vi "ao_waveform_pc_infinite.vi"() -> ()   [LabVIEW 2020]
uses:
  <vilib>/measure/NI_MABase.lvlib
panel:
  out "x-y":u32
  out "Rounds":i32
  out "error out":errorcluster caption="错误输出"
  in  "停止":bool
  out "波形图":waveform(dbl)(graph)
  in  "SamplePeriod (ns)":u32=10000
  in  "Chan":u8
  in  "DevIndex":i32
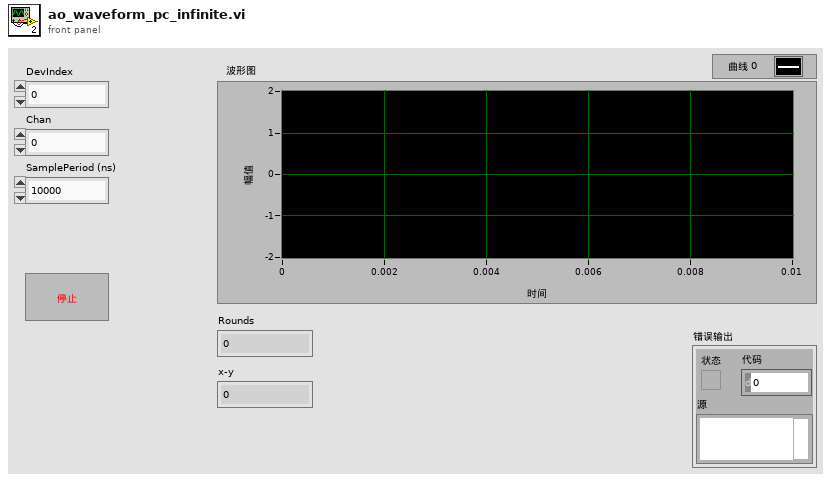
[diagram p1: front panel]
types:
  T1 = enum16{"Sine Wave", "Triangle Wave", "Square Wave", "Sawtooth Wave"}
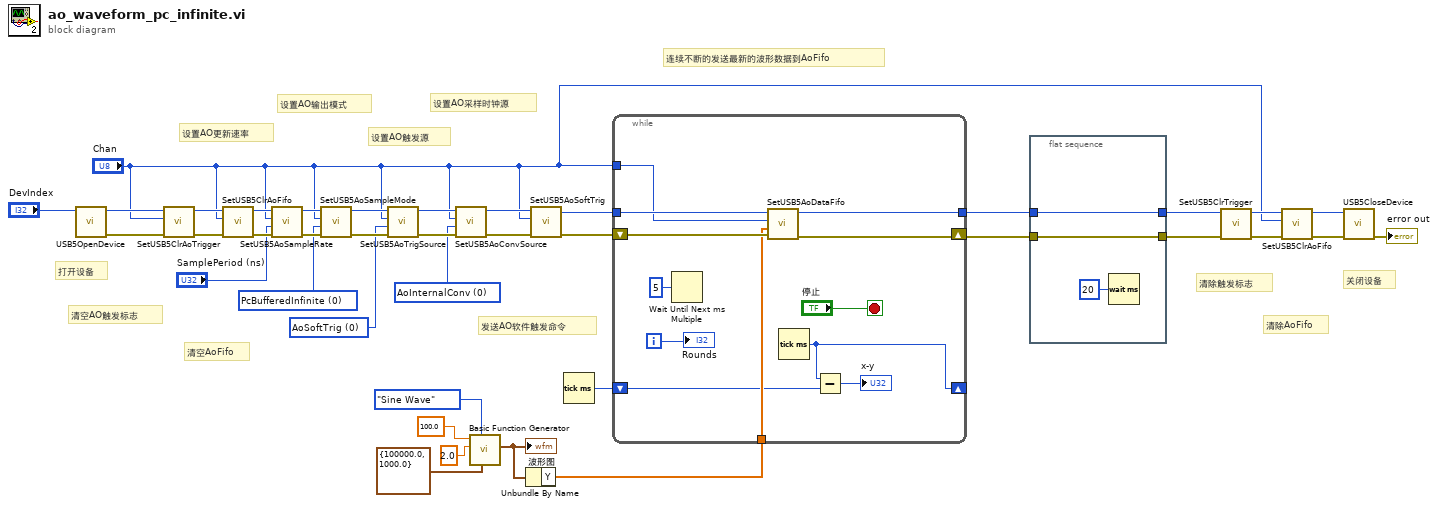
[diagram p0: block diagram]
diagram:
  w1 = u8 0 items=["AoInternalConv", "ConvIn", "AiConv", "DiConv", "DoConv", "Ao0Conv", "Ao1Conv", "Ao2Conv", "Ao3Conv"] ("AoConvSource")
  w2 = u8 0 items=["AoSoftTrig"=0, "ExtTrigIn"=1, "Din0RisingEdge"=2, "Din1RisingEdge"=3, "Din2RisingEdge"=4, "Din3RisingEdge"=5, "WithAiTrig"=6, "WithDiTrig"=7, "WithDoTrig"=8, "WithAo0Trig"=9, "WithAo1Trig"=10, "WithAo2Trig"=11, "WithAo3Trig"=12, "GlobalSoftTrig"=255] ("AoTrigSource")
  w3 = u8 0 items=["PcBufferedInfinite", "NCycle"] ("SampleMode")
  # "关闭设备"
  # "清除AoFifo"
  # "清除触发标志"
  # "连续不断的发送最新的波形数据到AoFifo"
  # "发送AO软件触发命令"
  # "设置AO采样时钟源"
  # "设置AO触发源"
  # "设置AO输出模式"
  # "设置AO更新速率"
  # "清空AoFifo"
  # "清空AO触发标志"
  # "打开设备"
  n1 = call "USB5OpenDevice.vi"("DevIndex"="DevIndex") -> ("error out"=w14:errorcluster, "DevIndex Out"=w15:i32)  [unwired: 9 in]
  n2 = call "SetUSB5ClrAoTrigger.vi"("错误输入（无错误）"=w14, "Chan"="Chan", "DevIndex"=w15) -> ("错误输出"=w12:errorcluster, "DevIndex Out"=w13:i32)  [unwired: 7 in]
  n3 = call "SetUSB5ClrAoFifo.vi"("错误输入（无错误）"=w12, "Chan"="Chan", "DevIndex"=w13) -> ("错误输出"=w32:errorcluster, "DevIndex Out"=w31:i32)  [unwired: 7 in]
  n4 = call "SetUSB5AoSampleRate.vi"("错误输入（无错误）"=w32, "SamplePeriod(ns)"="SamplePeriod (ns)", "Chan"="Chan", "DevIndex"=w31) -> ("错误输出"=w27:errorcluster, "DevIndex Out"=w28:i32)  [unwired: 6 in]
  n5 = call "SetUSB5AoSampleMode.vi"("错误输入（无错误）"=w27, "SampleMode"=w3, "Chan"="Chan", "DevIndex"=w28) -> ("错误输出"=w10:errorcluster, "DevIndex Out"=w11:i32)  [unwired: 6 in]
  n6 = call "SetUSB5AoTrigSource.vi"("错误输入（无错误）"=w10, "AoTrigSource"=w2, "Chan"="Chan", "DevIndex"=w11) -> ("错误输出"=w8:errorcluster, "DevIndex Out"=w9:i32)  [unwired: 6 in]
  n7 = call "SetUSB5AoConvSource.vi"("错误输入（无错误）"=w8, "AoConvSource"=w1, "Chan"="Chan", "DevIndex"=w9) -> ("错误输出"=w6:errorcluster, "DevIndex Out"=w7:i32)  [unwired: 6 in]
  n8 = call <vilib>:"Basic Function Generator.vi"("sampling info"=cluster{"Fs":dbl, "#s":dbl} {"Fs"=100000.0, "#s"=1000.0}, "signal type"=T1."Sine Wave", "amplitude"=2.0, "frequency"=100.0) -> ("signal out"=w34:waveform(dbl))  [unwired: 5 in, 2 out]
  "波形图" <- w34
  n9 = Unbundle By Name(w34) -> ("Y"=w33:dbl[])
  n10 = call "SetUSB5AoSoftTrig.vi"("错误输入（无错误）"=w6, "Chan"="Chan", "DevIndex"=w7) -> ("错误输出"=w25:errorcluster, "DevIndex Out"=w26:i32)  [unwired: 7 in]
  n11 = Tick Count (ms)() -> (millisecond timer value=w4:u32)
  n12 = while {
    tunnel: w26 -> [w50]
    tunnel: "Chan" -> [w48]
    tunnel: w33 -> [w46]
    tunnel: [w44] -> w18
    shift-right: [w43] -> w16
    shift-left: w25 -> [w49]
    shift-right: [w39] -> _
    shift-left: w4 -> [w41]
    i -> [w42]
    stop <- "停止" stop-if-true
    n13 = Wait Until Next ms Multiple(millisecond multiple=u32 5 ("毫秒倍数")) -> ()  [unwired: 1 out]
    n14 = call "SetUSB5AoDataFifo.vi"("错误输入（无错误）"=w49, "Voltage"=w46, "Chan"=w48, "DevIndex"=w50) -> ("错误输出"=w43:errorcluster, "DevIndex Out"=w44:i32)  [unwired: 6 in]
    n15 = Tick Count (ms)() -> (millisecond timer value=w39:u32)
    n16 = Subtract(x=w39, y=w41) -> (x-y=→"x-y":u32)
    "Rounds" <- w42
  }
  n17 = flat-sequence {
    tunnel: [w53] -> w19
    tunnel: w18 -> [w53]
    tunnel: [w52] -> w17
    tunnel: w16 -> [w52]
    frame #0 {
      n18 = Wait (ms)(milliseconds to wait=u32 20 ("等待时间（毫秒）")) -> ()  [unwired: 1 out]
    }
  }
  n19 = call "SetUSB5ClrTrigger.vi"("错误输入（无错误）"=w17, "DevIndex"=w19) -> ("错误输出"=w23:errorcluster, "DevIndex Out"=w24:i32)  [unwired: 8 in]
  n20 = call "SetUSB5ClrAoFifo.vi"("错误输入（无错误）"=w23, "Chan"="Chan", "DevIndex"=w24) -> ("错误输出"=w21:errorcluster, "DevIndex Out"=w22:i32)  [unwired: 7 in]
  n21 = call "USB5CloseDevice.vi"("错误输入（无错误）"=w21, "DevIndex"=w22) -> ("error out"=→"error out":errorcluster)  [unwired: 8 in, 1 out]
